vi "waypoint_icon_to_bitmap.vi"(8 "Index":i32, 9 "Done?":bool, 10 "Mission Waypoint?":bool, 11 "Waypoint Icon References":T1) -> (1 "Icon Bitmap Out":u32[][](array[colorbox]), 3 "Icon Out":T2(plugin-control))   [LabVIEW 2013]
doc: "Rotates icon images of the boat and sails and overlays them on each other to create a representation of the current state of the robot. Also converts the output image to a bitmap for easy overlay on the mission map.\n\norigininally by Jason Curtis\nAdapted 4/5/2014 by Mac-I Crowell"
uses:
  TypeDef/waypoint_icon_references.ctl
  <vilib>/vision/Image Controls.llb/IMAQ Image.ctl
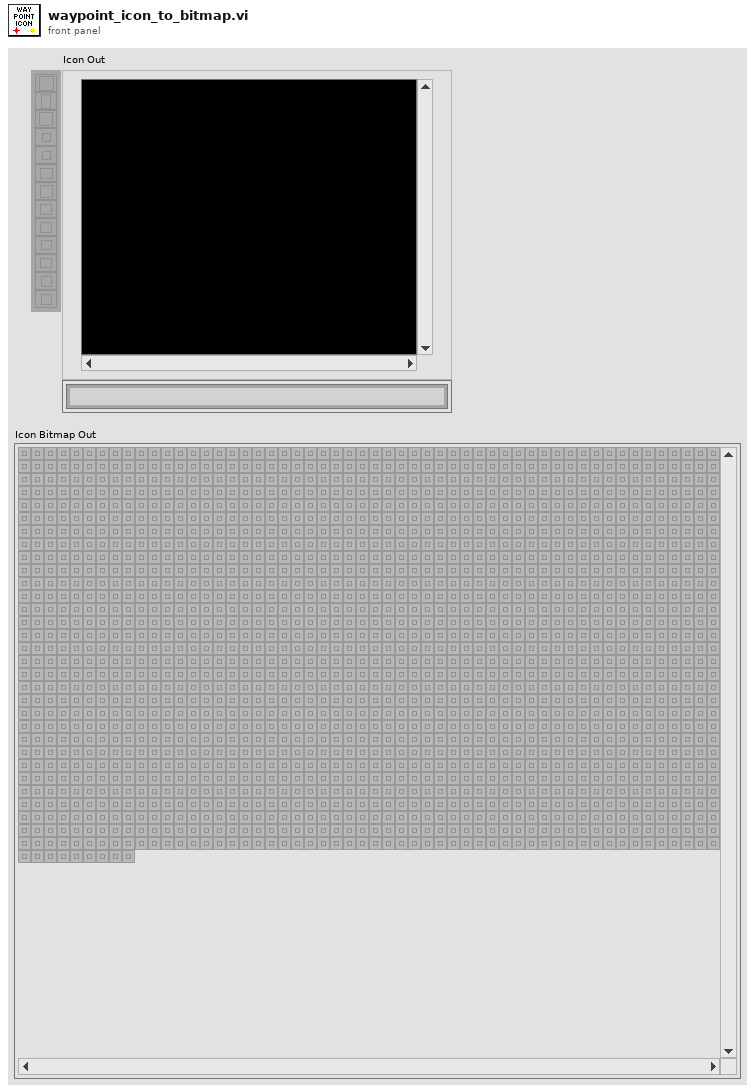
[diagram p1: front panel]
types:
  T1 = typedef "waypoint_icon_references.ctl" = cluster{"Mission Waypoint Icon":T2, "Sailing Point Icon":T2, "Mission Waypoint Done Icon":T2, "Sailing Point Done Icon":T2, "Next Mission Waypoint Icon":T2, "Next Sailing Point Icon":T2}
  T2 = typedef "IMAQ Image.ctl" = refnum<image>
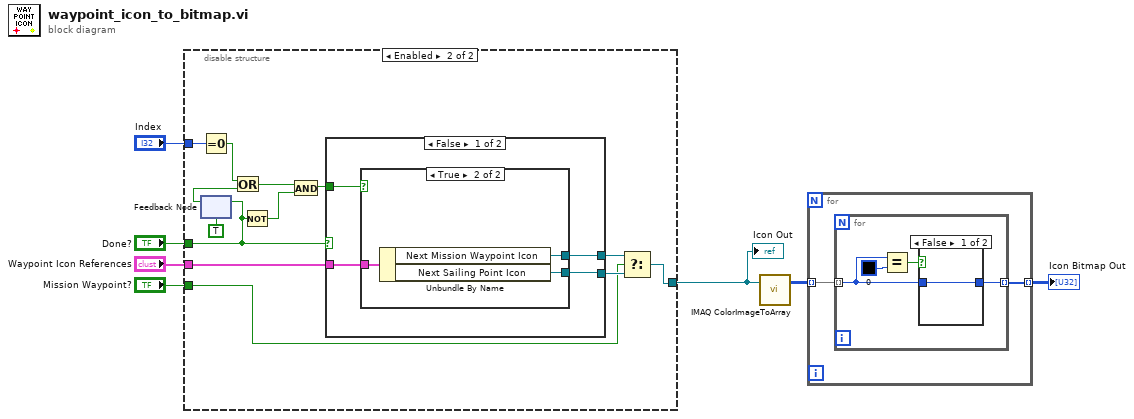
[diagram p0: block diagram]
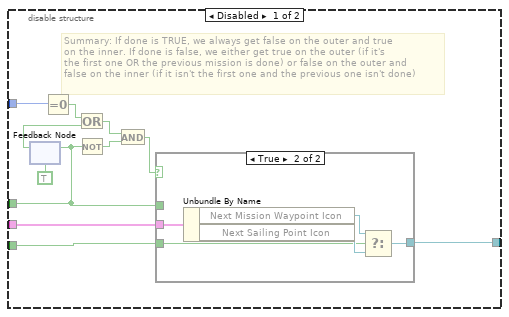
[diagram p2: hidden frame]
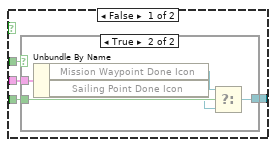
[diagram p3: hidden frame]
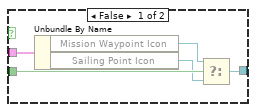
[diagram p4: hidden frame]
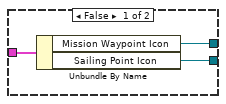
[diagram p5: hidden frame]
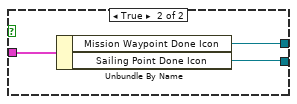
[diagram p6: hidden frame]
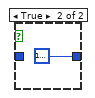
[diagram p7: hidden frame]
diagram:
  n1 = disable-structure shown="Enabled" {
    disable-tunnel: "Waypoint Icon References" -> [w18 w50]
    disable-tunnel: "Mission Waypoint?" -> [w17 w46]
    disable-tunnel: [w16 w45] -> w3
    disable-tunnel: "Done?" -> [w14 w41]
    disable-tunnel: "Index" -> [w9 w49]
    frame Disabled {
      # "Summary: If done is TRUE, we always get false on the outer and true\non the inner. If done is false, we either get true on the outer (if it's\nthe first one OR the previous mission is done) or false on the outer and\nfalse on the inner (if it isn't the first one and the previous one isn't done)"
      n2 = feedback #1(TRUE ("Done?")) -> (w11:bool)
      n3 = feedback-in #1(w14) -> ()
      n4 = Equal To 0?(x=w9) -> (x = 0?=w10:bool)
      n5 = Or(x=w10, y=w11) -> (x .or. y?=w12:bool)
      n6 = Not(x=w14) -> (.not. x?=w15:bool)
      n7 = And(x=w12, y=w15) -> (x .and. y?=w8:bool)
      n8 = case shown="True" w8 {
        tunnel: w18 -> [w22 w33]
        tunnel: w17 -> [w21 w34]
        tunnel: [w20 w36] -> w16
        tunnel: w14 -> [w19 _]
        frame False {
          n9 = case shown="True" w19 {
            tunnel: w22 -> [w26 w32]
            tunnel: w21 -> [w27 w31]
            tunnel: [w23 w28] -> w20
            frame False {
              n10 = Unbundle By Name(w26) -> ("Mission Waypoint Icon"=w25:T2, "Sailing Point Icon"=w24:T2)
              n11 = Select(t=w25, s=w27, f=w24) -> (s? t:f=w23:T2)
            }
            frame True {
              n12 = Unbundle By Name(w32) -> ("Mission Waypoint Done Icon"=w30:T2, "Sailing Point Done Icon"=w29:T2)
              n13 = Select(t=w30, s=w31, f=w29) -> (s? t:f=w28:T2)
            }
          }
        }
        frame True {
          n14 = Unbundle By Name(w33) -> ("Next Mission Waypoint Icon"=w37:T2, "Next Sailing Point Icon"=w35:T2)
          n15 = Select(t=w37, s=w34, f=w35) -> (s? t:f=w36:T2)
        }
      }
    }
    frame Enabled {
      n16 = Equal To 0?(x=w49) -> (x = 0?=w40:bool)
      n17 = feedback #2(TRUE) -> (w39:bool)
      n18 = feedback-in #2(w41) -> ()
      n19 = Or(x=w40, y=w39) -> (x .or. y?=w38:bool)
      n20 = Not(x=w41) -> (.not. x?=w43:bool)
      n21 = And(x=w38, y=w43) -> (x .and. y?=w44:bool)
      n22 = case shown="False" w41 {
        tunnel: w50 -> [w54 w63]
        tunnel: [w53 w62] -> w48
        tunnel: [w52 w61] -> w47
        tunnel: w44 -> [w51 _]
        frame False {
          n23 = case shown="True" w51 {
            tunnel: w54 -> [w57 w60]
            tunnel: [w56 w59] -> w53
            tunnel: [w55 w58] -> w52
            frame False {
              n24 = Unbundle By Name(w57) -> ("Mission Waypoint Icon"=w56:T2, "Sailing Point Icon"=w55:T2)
            }
            frame True {
              n25 = Unbundle By Name(w60) -> ("Next Mission Waypoint Icon"=w59:T2, "Next Sailing Point Icon"=w58:T2)
            }
          }
        }
        frame True {
          n26 = Unbundle By Name(w63) -> ("Mission Waypoint Done Icon"=w62:T2, "Sailing Point Done Icon"=w61:T2)
        }
      }
      n27 = Select(t=w48, s=w46, f=w47) -> (s? t:f=w45:T2)
    }
  }
  "Icon Out" <- w3
  n28 = call "IMAQ ColorImageToArray"("Image"=w3) -> ("Image Pixels (U32)"=w6:u32[][])  [unwired: 2 in, 3 out]
  n29 = for {
    tunnel: w6 -> [w65] mode=indexing
    tunnel: [w64] -> w7 mode=indexing
    n30 = for {
      tunnel: w65 -> [w67] mode=indexing
      tunnel: [w68] -> w64 mode=indexing
      n31 = Equal?(x=w67, y=u32 0) -> (x = y?=w69:bool)
      n32 = case shown="False" w69 {
        tunnel: [w70 u32 16777216] -> w68
        tunnel: w67 -> [w70 _]
        frame False {
        }
        frame True {
        }
      }
    }
  }
  "Icon Bitmap Out" <- w7
